vi "Gestion Bouton Main.vi"(8 "error in (no error)":errorcluster caption="entrée d'erreur (pas d'erreur)", 9 "cluster de sortie":T1, 10 "File et Queue":T2, 11 "Gestion Interface":refnum<vi>) -> (0 "error out":errorcluster caption="sortie d'erreur")   [LabVIEW 2020]
uses:
  File et notificateur/File et notification.ctl
  TypeDef/Data Event Sequenceur.ctl
  TypeDef/Liste Event Sequenceur.ctl
  TypeDef/Liste Fonction appelante.ctl
  Tache Generation Historique/Type DEF/Data Event Historique.ctl
  Tache Generation Historique/Type DEF/Liste Event Historique.ctl
  Type DEF/Commande Selection produit en cours.ctl
  TypeDef/Commande Variable Global.ctl
  Type DEF/Commande Variables Programme.ctl
  Type DEF/Commande tableau Resultat.ctl
  Instrument/BLE/Comande Variable Globale BLE.ctl
  Drivers/BLE/type_def/connection_status_bundle.ctl
  Drivers/BLE/type_def/address_type.ctl
  Type DEF/Commande Event Demande Op.ctl
  Type DEF/Commande Event Demande Autotest.ctl
  Type DEF/Commande Action Lecture RS Bridge.ctl
  Type DEF/Commande Event Saisie Op.ctl
  TypeDef/Liste fonction Saisie Operateur.ctl
  Type DEF/Commande Event Affiche Result.ctl
  Fonction/Shielding Box/Action.ctl
  TypeDef/Adresse IHM.ctl
panel:
  # "Application"
  # "Sequenceur"
  # "Data"
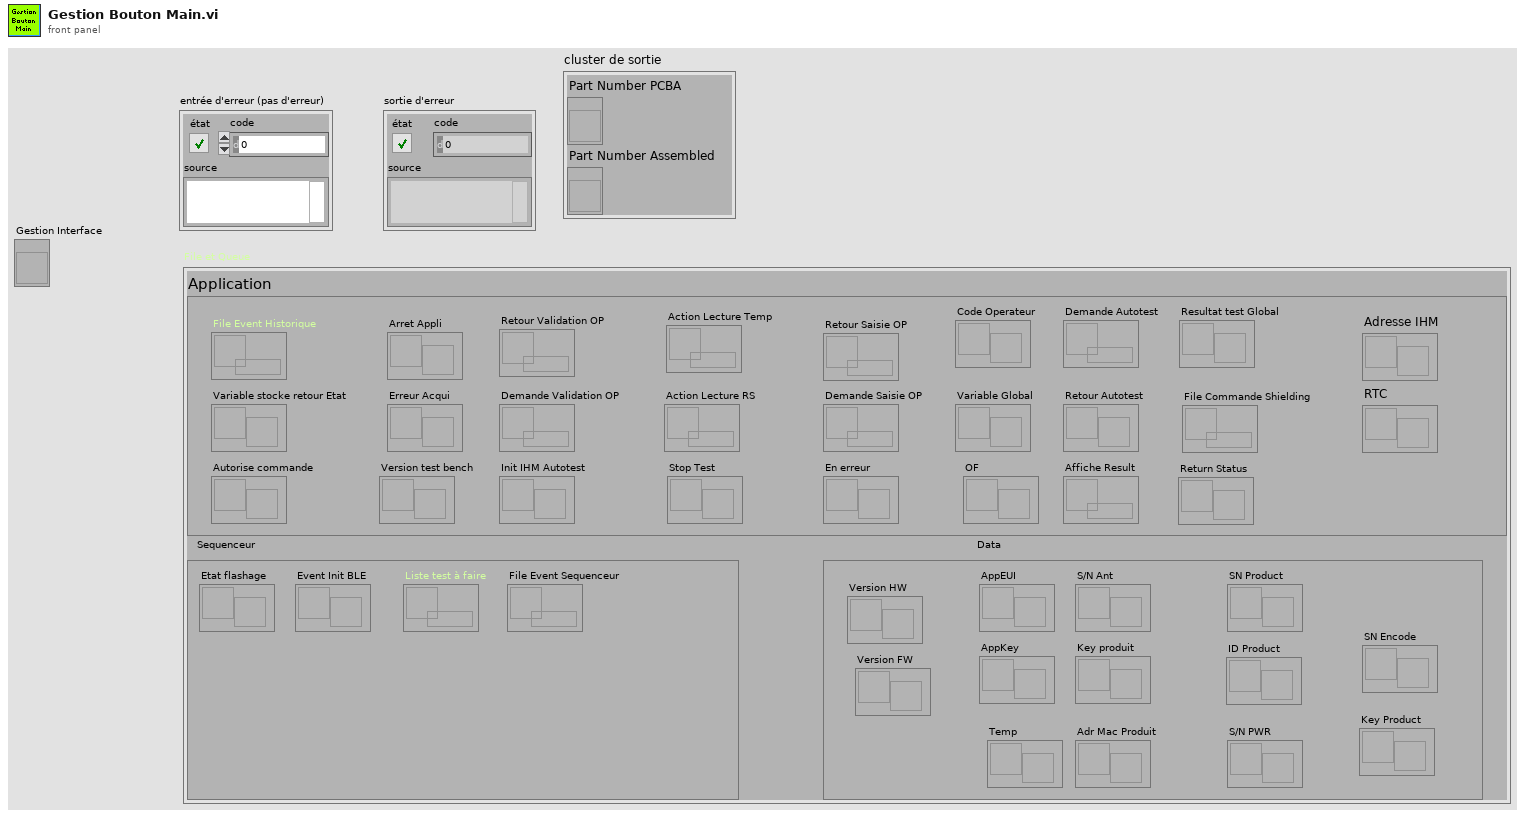
[diagram p1: front panel]
types:
  T1 = cluster{"Part Number PCBA":refnum<vi>, "Part Number Assembled":refnum<vi>}
  T2 = typedef "File et notification.ctl" = cluster{"Arret Appli":refnum<notifier>, "Erreur Acqui":refnum<notifier>, "File Event Sequenceur":refnum<queue>, "Liste test à faire":refnum<queue>, "File Event Historique":refnum<queue>, "Variable Global":refnum<notifier>, "Variable stocke retour Etat":refnum<notifier>, "Retour Validation OP":refnum<queue>, "Demande Validation OP":refnum<queue>, "Retour Autotest":refnum<notifier>, "Demande Autotest":refnum<queue>, "Adr Mac Produit":refnum<notifier>, "Autorise commande":refnum<notifier>, "Event Init BLE":refnum<notifier>, "Action Lecture RS":refnum<queue>, "Key produit":refnum<notifier>, "Retour Saisie OP":refnum<queue>, "Demande Saisie OP":refnum<queue>, "Etat flashage":refnum<notifier>, "Code Operateur":refnum<notifier>, "Resultat test Global":refnum<notifier>, "Stop Test":refnum<notifier>, "Init IHM Autotest":refnum<notifier>, "Version test bench":refnum<notifier>, "SN Product":refnum<notifier>, "En erreur":refnum<notifier>, "Affiche Result":refnum<queue>, "S/N PWR":refnum<notifier>, "AppEUI":refnum<notifier>, "Action Lecture Temp":refnum<queue>, "Temp":refnum<notifier>, "AppKey":refnum<notifier>, "OF":refnum<notifier>, "File Commande Shielding":refnum<queue>, "Return Status":refnum<notifier>, "ID Product":refnum<notifier>, "Version FW":refnum<notifier>, "Version HW":refnum<notifier>, "Adresse IHM":refnum<notifier>, "RTC":refnum<notifier>, "S/N Ant":refnum<notifier>, "SN Encode":refnum<notifier>, "Key Product":refnum<notifier>}
  T3 = typedef "CheckBox 2.ctl" = u16
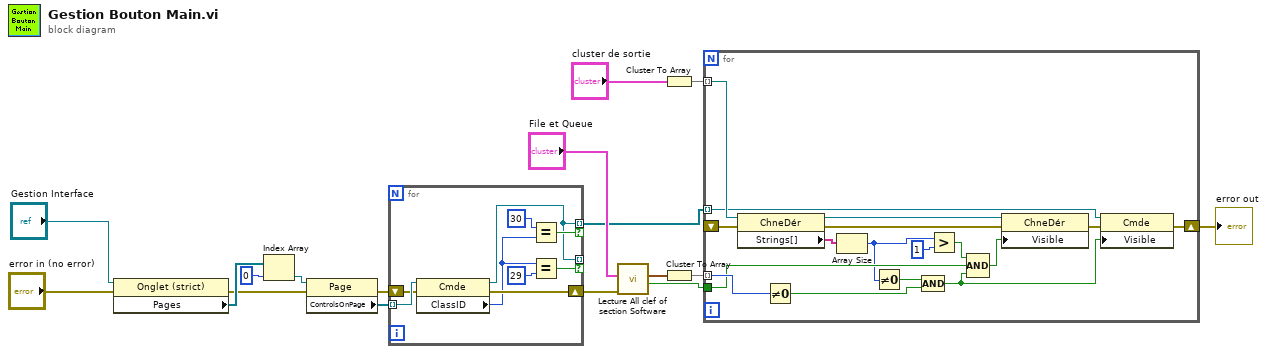
[diagram p0: block diagram]
diagram:
  n1 = property on="Nœud de propriété" class="Onglet (strict)"(reference="Gestion Interface", error in="error in (no error)") -> (error out=w9:errorcluster, "Pages"=w13:refnum<vi>[])  [unwired: 1 out]
  n2 = Index Array(array=w13, index=0 ("indice")) -> (element=w15:refnum<vi>)
  n3 = property class="Page"(reference=w15, error in=w9) -> (error out=w8:errorcluster, "ControlsOnPage"=w16:refnum<vi>[])  [unwired: 1 out]
  n4 = for {
    tunnel: w16 -> [w26] mode=indexing
    tunnel: [w19] -> w2 mode=indexing if=w25
    shift-right: [w22] -> w7
    shift-left: w8 -> [w23]
    tunnel: [w19] -> _ mode=indexing if=w18
    n5 = property class="Cmde"(reference=w26, error in=w23) -> (reference out=w19:refnum<vi>, error out=w22:errorcluster, "ClassID"=w21:u32)
    n6 = Equal?(x=u32 30, y=w21) -> (x = y?=w25:bool)
    n7 = Equal?(x=w21, y=u32 29) -> (x = y?=w18:bool)
  }
  n8 = call "Lecture All clef of section Software.vi"("error in (no error)"=w7, "File et Queue"="File et Queue") -> ("Multi Produit"=w5:bool, "Display"=w17:cluster{"CheckBox PCB":T3, "CheckBox PCBA":T3})  [unwired: 6 in, 2 out]
  n9 = Cluster To Array(cluster="cluster de sortie") -> (array=w6:refnum<vi>[])
  n10 = Cluster To Array(cluster=w17) -> (array=w1:T3[])
  n11 = for {
    tunnel: w6 -> [w42] mode=indexing
    shift-right: [w35] -> w4
    shift-left: _ -> [w40]
    tunnel: w5 -> [w32]
    tunnel: w2 -> [w33] mode=indexing
    tunnel: w1 -> [w34] mode=indexing
    n12 = property class="ChneDér"(reference=w42, error in=w40) -> (reference out=w38:refnum<vi>, error out=w39:errorcluster, "Strings[]"=w41:string[])
    n13 = Not Equal To 0?(x=w34) -> (x != 0?=w30:bool)
    n14 = Array Size(array=w41) -> (size(s)=w29:i32)
    n15 = Not Equal To 0?(x=w29) -> (x != 0?=w28:bool)
    n16 = Compound Arithmetic op=AND ("Opérateur arithmétique")(w28, w30) -> (w27:bool)
    n17 = Greater?(x=w29, y=1) -> (0:w31:bool)
    n18 = Compound Arithmetic op=AND ("Opérateur arithmétique")(w31, w32, w27) -> (w37:bool)
    n19 = property class="ChneDér"(reference=w38, error in=w39, "Visible"=w37) -> (error out=w36:errorcluster)  [unwired: 1 out]
    n20 = property class="Cmde"(reference=w33, error in=w36, "Visible"=w27) -> (error out=w35:errorcluster)  [unwired: 1 out]
  }
  "error out" <- w4
